vi "Dark Current Test with Manual Measurment.vi"() -> ()   [LabVIEW 2020]
uses:
  <instrlib>/CAEN PSM/CAEN PSM.lvlib
panel:
  in  "VISA resource name 2":refnum<visa-resource-name>
  in  "Channel #":i32
  out "Power Supply Trip":bool
  out "Time Left (s)":dbl
  out "8":bool
  out "7":bool
  out "6":bool
  out "5":bool
  out "4":bool
  out "3":bool
  out "2":bool
  out "1":bool
  out "Test is Running":bool
  in  "Begin Test":bool
  out "Manual Measurments \nNeeded":bool
  out "OVV? 2":bool=TRUE
  out "OVC? 2":bool=TRUE
  out "Actual Voltage Level (V) 2":dbl format="%#_13g"
  out "Recorded Current\nfor Previous Tube":dbl format="%#_13g"
  in  "Measure Next Tube":bool
  in  "Barcodes":string[](array[string])
  out "Next Measurment":string
  in  "N":i32
  in  "dt (s)":i32
  out "Actual Current Limit (nA)":dbl format="%#_13g"
  out "Actual Voltage Level (V)":dbl format="%#_13g"
  out "OVC?":bool=TRUE
  out "OVV?":bool=TRUE
  # "Dark Current Test"
  # "Instructions in Brief:\n1. Begin the program by clicking the white arrow.\n2. Assemble tubes into the test bench.\n3. Select COM5 for the \"VISA resource name\".\n4. Enter in how often you want to take measurement in the \"dt\" box (typically 60s)\n5. Enter in how many measurments you want to take (typically 15)\n6. Scan in the 8 tubes that you are testing.\n(If you take 15 measurments every 60s, the test will take 15 min.)\n7. Click \"Begin Test\". The \"Test is Running\" LED should light up.\n8. After the intial test, if the total current is below 16nA, \n    the program will write the \n     file and end the test.\n9. If the total current is above 16nA, manual\n    measurments need to be taken.\n10. Engage only the tube indicated by \"Next Measurment\". \n11. Click \"Measure\".\n12. Engage the next tube and continue untill all have been measured.\n13. In both cases, the program will write files and end the test. \n14. The test is over when the \"Test is Running\" LED has turned off."
  # "Green lights indicate tubes that have passed."
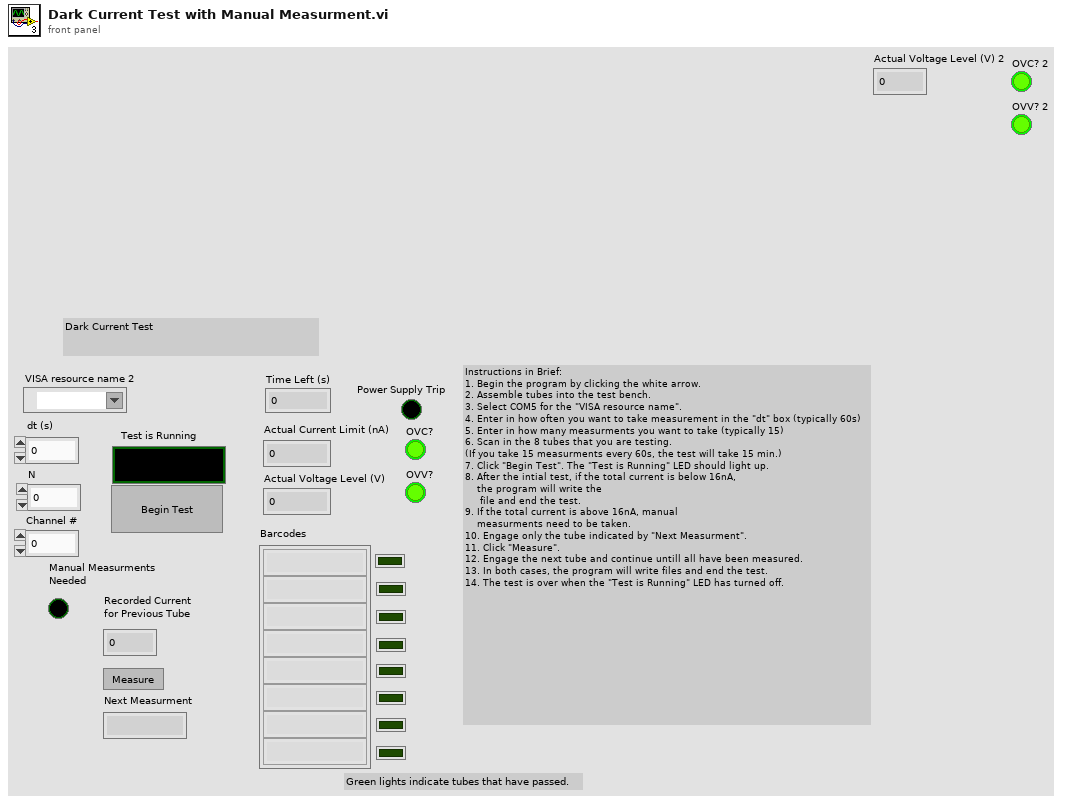
[diagram p1: front panel]
types:
  T1 = cluster{"VISA resource name":refnum<visa-resource-name>, "Board address":u8, "NChannels":u8}
  T2 = cluster{"ON":bool, "RUP":bool, "RDW":bool, "OVC":bool, "OVV":bool, "UNV":bool, "MAXV":bool, "TRIP":bool, "OVP":bool, "OVT":bool, "DIS":bool, "KILL":bool, "ILK":bool, "NOCAL":bool}[]
  T3 = cluster{"ON":bool, "RUP":bool, "RDW":bool, "OVC":bool, "OVV":bool, "UNV":bool, "MAXV":bool, "TRIP":bool, "OVP":bool, "OVT":bool, "DIS":bool, "KILL":bool, "ILK":bool, "NOCAL":bool}
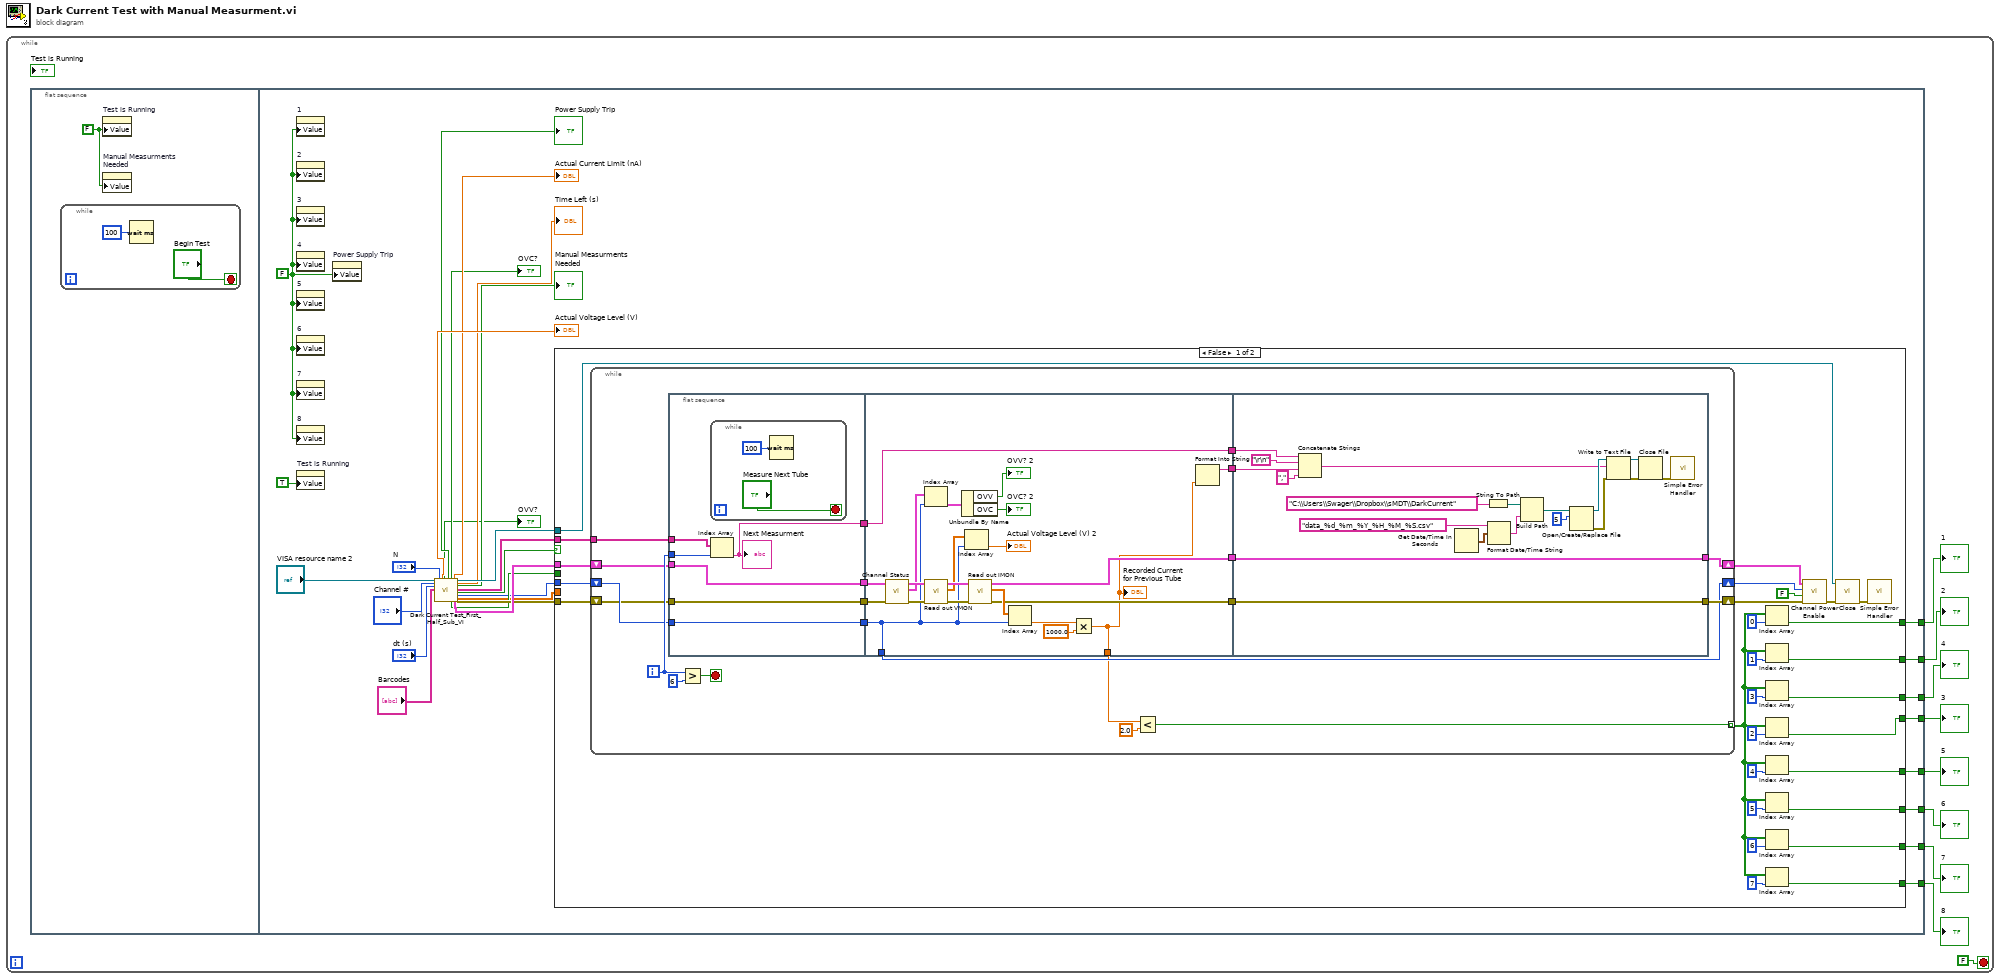
[diagram p0: block diagram]
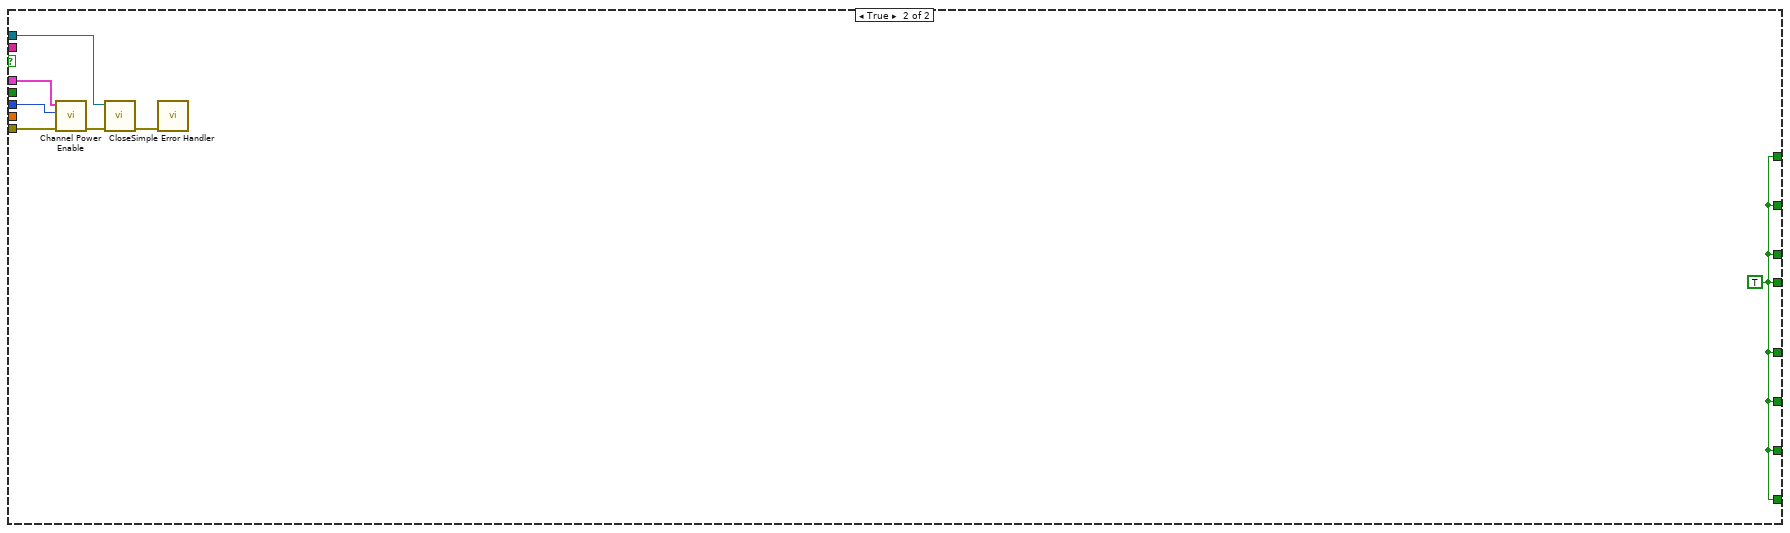
[diagram p2: hidden frame]
diagram:
  n1 = while {
    stop <- FALSE stop-if-true
    n2 = flat-sequence {
      tunnel: [w35] -> w8
      tunnel: [w34] -> w7
      tunnel: [w33] -> w6
      tunnel: [w32] -> w5
      tunnel: [w31] -> w4
      tunnel: [w30] -> w3
      tunnel: [w29] -> w2
      tunnel: [w28] -> w1
      frame #0 {
        w10 = FALSE
        n3 = while {
          stop <- "Begin Test" stop-if-true
          n4 = Wait (ms)(milliseconds to wait=100) -> ()  [unwired: 1 out]
        }
        n5 = property on="Test is Running" class="Bool (strict)"("Value"=w10) -> ()  [unwired: 2 in, 2 out]
        n6 = property on="Manual Measurments \nNeeded" class="Bool (strict)"("Value"=w10) -> ()  [unwired: 2 in, 2 out]
      }
      frame #1 {
        w26 = FALSE
        n7 = property on="1" class="Bool (strict)"("Value"=w26) -> ()  [unwired: 2 in, 2 out]
        n8 = property on="2" class="Bool (strict)"("Value"=w26) -> ()  [unwired: 2 in, 2 out]
        n9 = property on="3" class="Bool (strict)"("Value"=w26) -> ()  [unwired: 2 in, 2 out]
        n10 = property on="4" class="Bool (strict)"("Value"=w26) -> ()  [unwired: 2 in, 2 out]
        n11 = property on="5" class="Bool (strict)"("Value"=w26) -> ()  [unwired: 2 in, 2 out]
        n12 = property on="6" class="Bool (strict)"("Value"=w26) -> ()  [unwired: 2 in, 2 out]
        n13 = property on="7" class="Bool (strict)"("Value"=w26) -> ()  [unwired: 2 in, 2 out]
        n14 = property on="8" class="Bool (strict)"("Value"=w26) -> ()  [unwired: 2 in, 2 out]
        n15 = property on="Test is Running" class="Bool (strict)"("Value"=TRUE) -> ()  [unwired: 2 in, 2 out]
        n16 = property on="Power Supply Trip" class="Bool (strict)"("Value"=w26) -> ()  [unwired: 2 in, 2 out]
        n17 = call "Dark Current Test_First_Half_Sub_VI.vi"("VISA Refnum in"="VISA resource name 2", "Channel #"="Channel #", "dt (s)"="dt (s)", "Barcodes in"="Barcodes", "N"="N") -> ("Actual Voltage Level (V)"=→"Actual Voltage Level (V)":dbl, "OVV?"=→"OVV?":bool, "Power Supply Trip"=→"Power Supply Trip":bool, "OVC?"=→"OVC?":bool, "Boolean 2"=w39:bool, "Actual Current Limit (nA)"=→"Actual Current Limit (nA)":dbl, "BoardHandle out 2"=w41:T1, "VISA Refnum out"=w23:refnum<visa-resource-name>, "Time Left (s)"=→"Time Left (s)":dbl, "Manual Measurments \nNeeded"=→"Manual Measurments \nNeeded":bool, "Barcodes out"=w25:string[], "Boolean"=w37:bool, "Channel # 3"=w38:i32, "Array"=w27:dbl[], "error out"=w40:errorcluster)  [unwired: 8 in]
        n18 = case shown="False" w37 {
          tunnel: w41 -> [w69 w142]
          tunnel: w40 -> [w70 w141]
          tunnel: w39 -> [_ _]
          tunnel: w38 -> [w68 w140]
          tunnel: w23 -> [w64 w143]
          tunnel: w27 -> [_ _]
          tunnel: w25 -> [w60 _]
          tunnel: [w50 w146] -> w35
          tunnel: [w49 w146] -> w34
          tunnel: [w48 w146] -> w33
          tunnel: [w47 w146] -> w32
          tunnel: [w46 w146] -> w31
          tunnel: [w45 w146] -> w30
          tunnel: [w44 w146] -> w29
          tunnel: [w43 w146] -> w28
          frame False {
            n19 = while {
              shift-right: [w76] -> w61
              shift-left: w68 -> [w86]
              shift-right: [w78] -> w63
              shift-left: w69 -> [w83]
              shift-right: [w77] -> w62
              shift-left: w70 -> [w81]
              tunnel: w60 -> [w74]
              tunnel: [w71] -> w59 mode=indexing
              i -> [w89]
              stop <- w90 stop-if-true
              n20 = flat-sequence {
                tunnel: w89 -> [w97]
                tunnel: [w96] -> w88
                tunnel: w86 -> [w95]
                tunnel: [w95] -> w85
                tunnel: [w94] -> w84
                tunnel: w83 -> [w94]
                tunnel: [w93] -> w82
                tunnel: w81 -> [w93]
                tunnel: w74 -> [w92]
                tunnel: w88 -> [w107]
                tunnel: [w107] -> w87
                tunnel: w85 -> [w102]
                tunnel: w84 -> [w105]
                tunnel: w82 -> [w106]
                tunnel: [w104] -> w80
                tunnel: [w103] -> w79
                tunnel: [w102] -> w76
                tunnel: [w101] -> w75
                tunnel: [w100] -> w73
                tunnel: w87 -> [w125]
                tunnel: w80 -> [w123]
                tunnel: w79 -> [w122]
                tunnel: [w123] -> w78
                tunnel: [w122] -> w77
                tunnel: w75 -> [w121]
                frame #0 {
                  n21 = while {
                    stop <- "Measure Next Tube" stop-if-true
                    n22 = Wait (ms)(milliseconds to wait=100) -> ()  [unwired: 1 out]
                  }
                  n23 = Index Array(array=w92, index=w97) -> (element=w96:string)
                  "Next Measurment" <- w96
                }
                frame #1 {
                  n24 = call <instrlib>:"Channel Status.vi"("error in (no error)"=w106, "BoardHandle"=w105) -> ("error out"=w113:errorcluster, "Channel Status Array"=w109:T2, "BoardHandle out"=w114:T1)  [unwired: 7 in]
                  n25 = Index Array(array=w109, index=w102) -> (element=w110:T3)
                  n26 = call <instrlib>:"Read out VMON.vi"("error in (no error)"=w113, "BoardHandle"=w114) -> ("error out"=w117:errorcluster, "VMon values (V)"=w115:dbl[], "BoardHandle out"=w116:T1)  [unwired: 7 in]
                  n27 = Unbundle By Name(w110) -> ("OVV"=→"OVV? 2":bool, "OVC"=→"OVC? 2":bool)
                  n28 = Index Array(array=w115, index=w102) -> (element=→"Actual Voltage Level (V) 2":dbl)
                  n29 = call <instrlib>:"Read out IMON.vi"("error in (no error)"=w117, "BoardHandle"=w116) -> ("error out"=w103:errorcluster, "IMon values (uA)"=w120:dbl[], "BoardHandle out"=w104:T1)  [unwired: 6 in, 1 out]
                  n30 = Index Array(array=w120, index=w102) -> (element=w118:dbl)
                  n31 = Multiply(x=w118, y=1000.0) -> (x*y=w100:dbl)
                  "Recorded Current\nfor Previous Tube" <- w100
                  n32 = Format Into String(w100) -> (resulting string=w101:string)  [unwired: 3 in, 1 out]
                }
                frame #2 {
                  n33 = Concatenate Strings(w125, "\r\n", w121, ",") -> (w127:string)
                  n34 = Get Date/Time In Seconds() -> (seconds since 1Jan1904=w137:timestamp)
                  n35 = String To Path(string="C:\\Users\\Swager\\Dropbox\\sMDT\\DarkCurrent") -> (path=w136:path)
                  n36 = Format Date/Time String(time format string (%c)="data_%d_%m_%Y_%H_%M_%S.csv", seconds (now)=w137) -> (date/time string=w138:string)  [unwired: 1 in]
                  n37 = Build Path(base path=w136, name or relative path=w138) -> (appended path=w134:path)
                  n38 = Open/Create/Replace File(file path (use dialog)=w134, operation (0:open)=5) -> (refnum out=w133:refnum<file>, error out=w132:errorcluster)  [unwired: 4 in, 1 out]
                  n39 = Write to Text File(file (use dialog)=w133, text=w127, error in=w132) -> (refnum out=w131:refnum<file>, error out=w130:errorcluster)  [unwired: 1 in, 1 out]
                  n40 = Close File(refnum=w131, error in=w130) -> (error out=w129:errorcluster)  [unwired: 1 out]
                  n41 = call <vilib>:"Simple Error Handler.vi"("error in (no error)"=w129) -> ()  [unwired: 4 in, 5 out]
                }
              }
              n42 = Greater?(x=w89, y=6) -> (0:w90:bool)
              n43 = Less?(x=w73, y=2.0) -> (x < y?=w71:bool)
            }
            n44 = Index Array(array=w59, index=0) -> (element=w50:bool)
            n45 = Index Array(array=w59, index=1) -> (element=w49:bool)
            n46 = Index Array(array=w59, index=3) -> (element=w47:bool)
            n47 = Index Array(array=w59, index=2) -> (element=w48:bool)
            n48 = Index Array(array=w59, index=4) -> (element=w46:bool)
            n49 = Index Array(array=w59, index=5) -> (element=w45:bool)
            n50 = Index Array(array=w59, index=6) -> (element=w44:bool)
            n51 = Index Array(array=w59, index=7) -> (element=w43:bool)
            n52 = call <instrlib>:"Channel Power Enable.vi"("error in (no error)"=w62, "Enable (OFF)"=FALSE, "Channel (0)"=w61, "BoardHandle"=w63) -> ("error out"=w66:errorcluster)  [unwired: 6 in, 1 out]
            n53 = call <instrlib>:"Close.vi"("error in (no error)"=w66, "VISA resource name"=w64) -> ("error out"=w65:errorcluster)  [unwired: 9 in]
            n54 = call <vilib>:"Simple Error Handler.vi"("error in (no error)"=w65) -> ()  [unwired: 4 in, 5 out]
          }
          frame True {
            w146 = TRUE
            n55 = call <instrlib>:"Channel Power Enable.vi"("error in (no error)"=w141, "Channel (0)"=w140, "BoardHandle"=w142) -> ("error out"=w145:errorcluster)  [unwired: 7 in, 1 out]
            n56 = call <instrlib>:"Close.vi"("error in (no error)"=w145, "VISA resource name"=w143) -> ("error out"=w144:errorcluster)  [unwired: 9 in]
            n57 = call <vilib>:"Simple Error Handler.vi"("error in (no error)"=w144) -> ()  [unwired: 4 in, 5 out]
          }
        }
      }
    }
    "1" <- w8
    "2" <- w7
    "3" <- w6
    "4" <- w5
    "5" <- w4
    "8" <- w1
    "6" <- w3
    "7" <- w2
  }
